vi "Set Color.vi"(8 "error in (no error)":errorcluster, 10 "Color Message.lvclass":refnum<class "Color Message.lvclass">, 11 "Table View in":refnum<class "Table View.lvclass">) -> (0 "error out":errorcluster, 3 "Table View out":refnum<class "Table View.lvclass">)   [LabVIEW 2020, in "[V]Table View.lvlib" / "Table View.lvclass"]
uses:
  Table View.lvclass
  Color Interface/Color/Color Message.lvclass
  Table View.lvclass/Table View.ctl
  Color Interface/Color/Color Message.lvclass/Color Message.ctl
  Color Interface/Color/Accessors/Read BG Color.vi
  Color Interface/Color/Accessors/Read txt Color.vi
  <vilib>/HUASUI/MulListBox/MListBox.lvclass
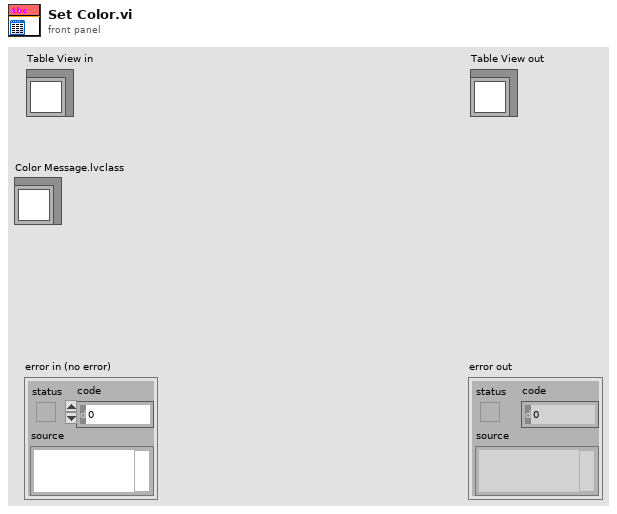
[diagram p1: front panel]
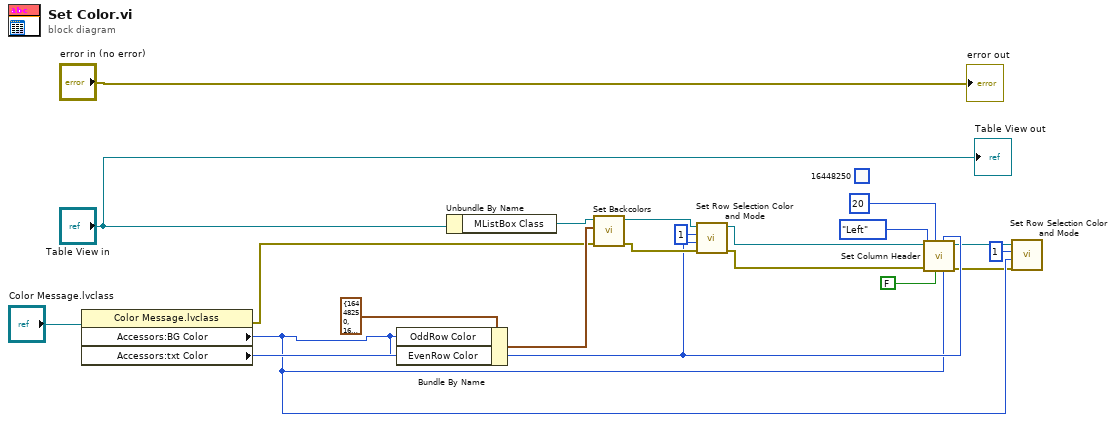
[diagram p0: block diagram]
diagram:
  (unwired) u32 16448250 ("Font Color")
  n1 = property class="Color Message.lvclass"(reference="Color Message.lvclass") -> (error out=w12:errorcluster, "Accessors:BG Color"=w2:u32, "Accessors:txt Color"=w5:u32)  [unwired: 1 in, 1 out]
  n2 = Bundle By Name(cluster=cluster{"OddRow Color":u32, "EvenRow Color":u32} {"OddRow Color"=16448250, "EvenRow Color"=16448250} ("BackColors"), "OddRow Color"=w2, "EvenRow Color"=w2) -> (w13:cluster{"OddRow Color":u32, "EvenRow Color":u32})
  n3 = Unbundle By Name("Table View in") -> ("MListBox Class"=w15:refnum<class "MListBox.lvclass">)
  n4 = call <vilib>:"Set Backcolors.vi"("error in (no error)"=w12, "BackColors"=w13, "Multicolumn ListBox in"=w15) -> ("error out"=w11:errorcluster, "Multicolumn ListBox out"=w14:refnum<class "MListBox.lvclass">)  [unwired: 7 in]
  n5 = call <vilib>:"Set Row Selection Color and Mode.vi"("error in (no error)"=w11, "Selected Color"=w5, "Selection Mode"=1, "Multicolumn ListBox in"=w14) -> ("error out"=w6:errorcluster, "Multicolumn ListBox out"=w7:refnum<class "MListBox.lvclass">)  [unwired: 6 in]
  n6 = call <vilib>:"Set Column Header.vi"("BackColor"=w2, "Font Color"=w5, "Active Cell:Cell Font:Bold"=FALSE, "Font:Size"=u32 20, "error in (no error)"=w6, "Justification"=enum16{"Left", "Center", "Right"}."Left", "Multicolumn ListBox in"=w7) -> ("error out"=w1:errorcluster, "Multicolumn ListBox out"=w4:refnum<class "MListBox.lvclass">)  [unwired: 3 in]
  n7 = call <vilib>:"Set Row Selection Color and Mode.vi"("error in (no error)"=w1, "Selected Color"=w2, "Selection Mode"=1, "Multicolumn ListBox in"=w4) -> ()  [unwired: 6 in, 2 out]
  "error out" <- "error in (no error)"
  "Table View out" <- "Table View in"
